vi "lib Overwrite Error.vi"(7 "Force Error?":bool, 8 "error in (no error)":errorcluster, 9 "Append Original Error Source?":bool, 10 "code":i32, 11 "Error Message":string) -> (0 "error out":errorcluster)   [LabVIEW 2021]
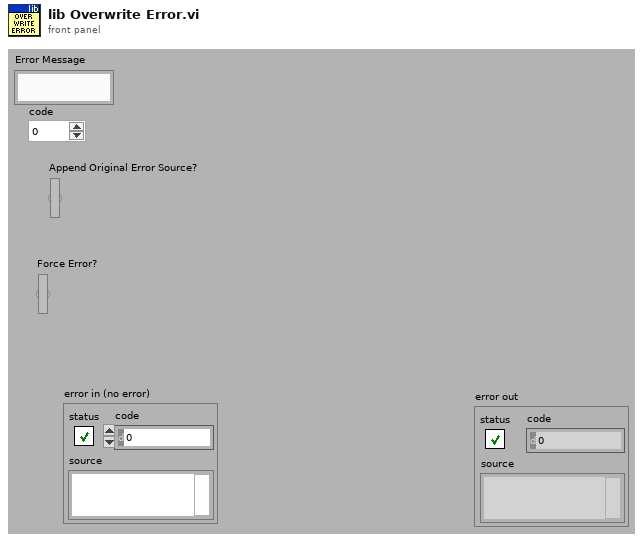
[diagram p1: front panel]
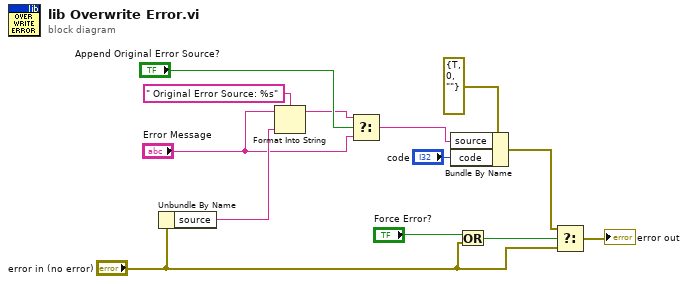
[diagram p0: block diagram]
diagram:
  n1 = Unbundle By Name("error in (no error)") -> ("source"=w8:string)
  n2 = Format Into String(format string=" Original Error Source: %s", initial string="Error Message", w8) -> (resulting string=w6:string)  [unwired: 1 in, 1 out]
  n3 = Select(t=w6, s="Append Original Error Source?", f="Error Message") -> (s? t:f=w4:string)
  n4 = Bundle By Name(cluster=errorcluster {"status"=TRUE, "code"=0, "source"=""} ("error in (no error)"), "source"=w4, "code"="code") -> (w10:errorcluster)
  n5 = Or(x="Force Error?", y="error in (no error)") -> (x .or. y?=w1:bool)
  n6 = Select(t=w10, s=w1, f="error in (no error)") -> (s? t:f=→"error out":errorcluster)
